vi "Write sampling.vi"(8 "error in (no error)":errorcluster, 10 "sampling":T1={"Fs"=204789.0, "#s"=15753}, 11 "Instrument.Lockin in":refnum<class "Instrument.Lockin.lvclass">) -> (0 "error out":errorcluster, 3 "Instrument.Lockin out":refnum<class "Instrument.Lockin.lvclass">)   [LabVIEW 2016, in "Instrument.Lockin.lvclass"]
uses:
  Instrument.Lockin.lvclass
  LockinDAQ/Typedefs/Sampling.ctl
  LockinDAQ/LockinDAQ.lvclass
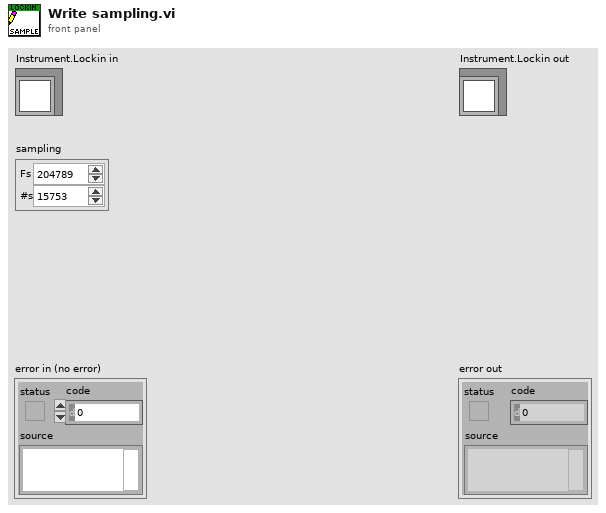
[diagram p1: front panel]
types:
  T1 = typedef "LockinDAQ.lvclass/Sampling.ctl" = cluster{"Fs":dbl, "#s":i32}
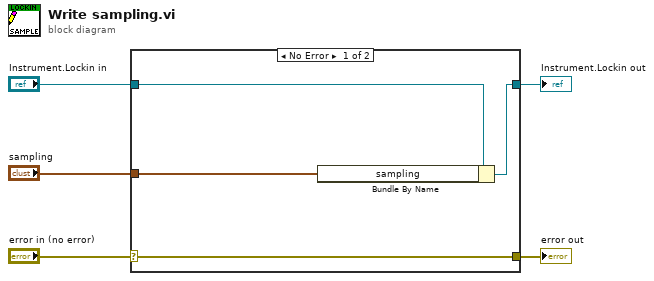
[diagram p0: block diagram]
diagram:
  n1 = case shown="No Error" "error in (no error)" {
    selector: "error in (no error)" -> [w9 w10]
    tunnel: [w9 w10] -> w4
    tunnel: [w7 w11] -> w2
    tunnel: "Instrument.Lockin in" -> [w8 w11]
    tunnel: "sampling" -> [w6 _]
    frame No Error {
      n2 = Bundle By Name(cluster=w8, "sampling"=w6) -> (w7:refnum<class "Instrument.Lockin.lvclass">)
    }
    frame Error {
    }
  }
  "error out" <- w4
  "Instrument.Lockin out" <- w2
